vi "From Boolean.vi"(0 "Value":bool, 1 "Key":string) -> (2 "Map":refnum<class "Map.lvclass">)   [LabVIEW 2018, in "Toolkit.lvlib" / "Data.lvlib" / "Map.lvclass"]
uses:
  Map.lvclass
  Map.lvclass/Map.ctl
  Boolean/Boolean.lvclass
  D:/Users/cfield/Code/Field R&D Services/Mustache/LabVIEW/trunk/src/Toolkit/Data/Datum/Datum.lvclass
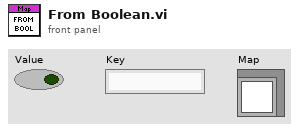
[diagram p1: front panel]
types:
  T1 = cluster{"Key":string, "Boolean":refnum<class "Boolean.lvclass">}
  T2 = cluster{"Key":string, "Boolean":refnum<class "Boolean.lvclass">}[]
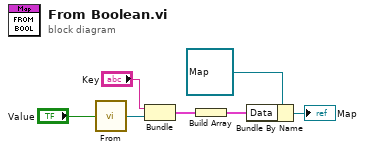
[diagram p0: block diagram]
diagram:
  n1 = call "From.vi"("Value"="Value") -> ("Boolean"=w1:refnum<class "Boolean.lvclass">)
  n2 = Bundle("Key"="Key", "Boolean"=w1) -> (w4:T1)  [unwired: 1 in]
  n3 = Build Array(w4) -> (w3:T2)
  n4 = Bundle By Name(cluster=refnum<class "Map.lvclass"> refnum ("Toolkit.lvlib:Data.lvlib:Map.lvclass"), "Data"=w3) -> (→"Map":refnum<class "Map.lvclass">)
